vi "DeleteChanGrp.vi"(8 "error in":errorcluster, 10 "ChanGroup":i32, 11 "TimingGrp in":refnum<class "TimingGrp.lvclass">) -> (0 "error out":errorcluster, 2 "ChanGrp.lvclass":refnum<class "ChanGrp.lvclass">, 3 "TimingGrp in":refnum<class "TimingGrp.lvclass">)   [LabVIEW 2018, in "Configuration Grandmaster.lvlib" / "TimingGrp.lvclass"]
uses:
  TimingGrp.lvclass
  Class Chan Group/ChanGrp.lvclass
  TimingGrp.lvclass/TimingGrp.ctl
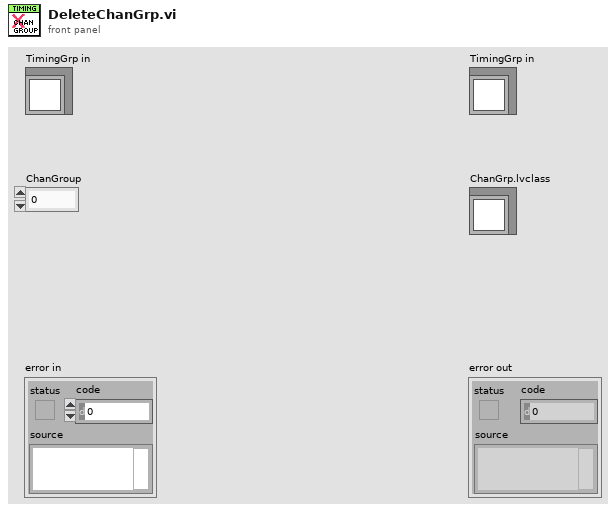
[diagram p1: front panel]
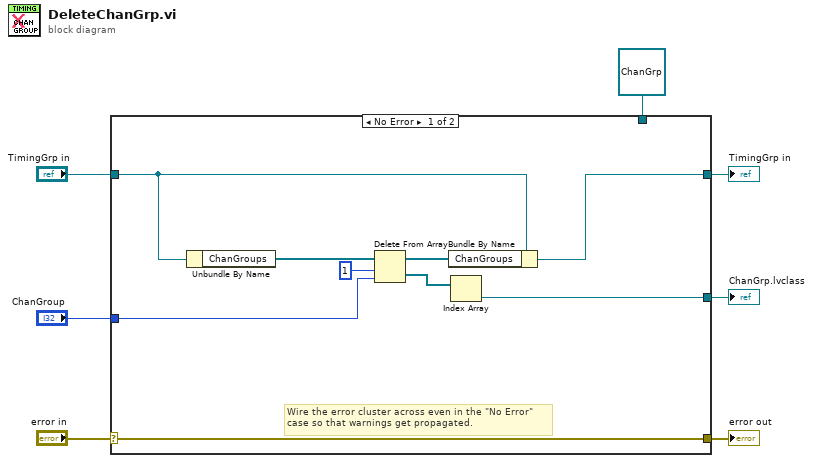
[diagram p0: block diagram]
diagram:
  n1 = case shown="No Error" "error in" {
    selector: "error in" -> [w16 w19]
    tunnel: [w16 w19] -> w6
    tunnel: [w10 w18] -> w4
    tunnel: "TimingGrp in" -> [w11 w18]
    tunnel: "ChanGroup" -> [w13 _]
    tunnel: [w8 w17] -> w2
    tunnel: refnum<class "ChanGrp.lvclass"> refnum ("GroupChans.lvclass") -> [_ w17]
    frame No Error {
      # "Wire the error cluster across even in the \"No Error\"\ncase so that warnings get propagated."
      n2 = Unbundle By Name(w11) -> ("ChanGroups"=w14:refnum<class "ChanGrp.lvclass">[])
      n3 = Delete From Array(array=w14, length=1, index=w13) -> (deleted portion=w9:refnum<class "ChanGrp.lvclass">[], array with subset deleted=w12:refnum<class "ChanGrp.lvclass">[])
      n4 = Bundle By Name(cluster=w11, "ChanGroups"=w12) -> (w10:refnum<class "TimingGrp.lvclass">)
      n5 = Index Array(array=w9) -> (element=w8:refnum<class "ChanGrp.lvclass">)  [unwired: 1 in]
    }
    frame Error {
    }
  }
  "error out" <- w6
  "TimingGrp in" <- w4
  "ChanGrp.lvclass" <- w2
